vi "gpibListener.vi"() -> ()   [LabVIEW 2011]
panel:
  in  "stop":bool
  out "Error Code":i32
  out "Error Status":bool
  out "Error Source":string
  in  "VISA resource name":refnum<visa-resource-name>
  out "Read Value":string
  out "Bytes Read":dbl
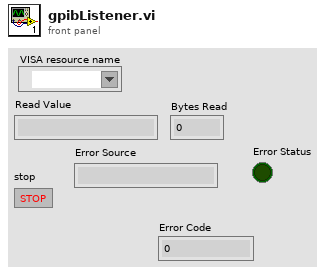
[diagram p1: front panel]
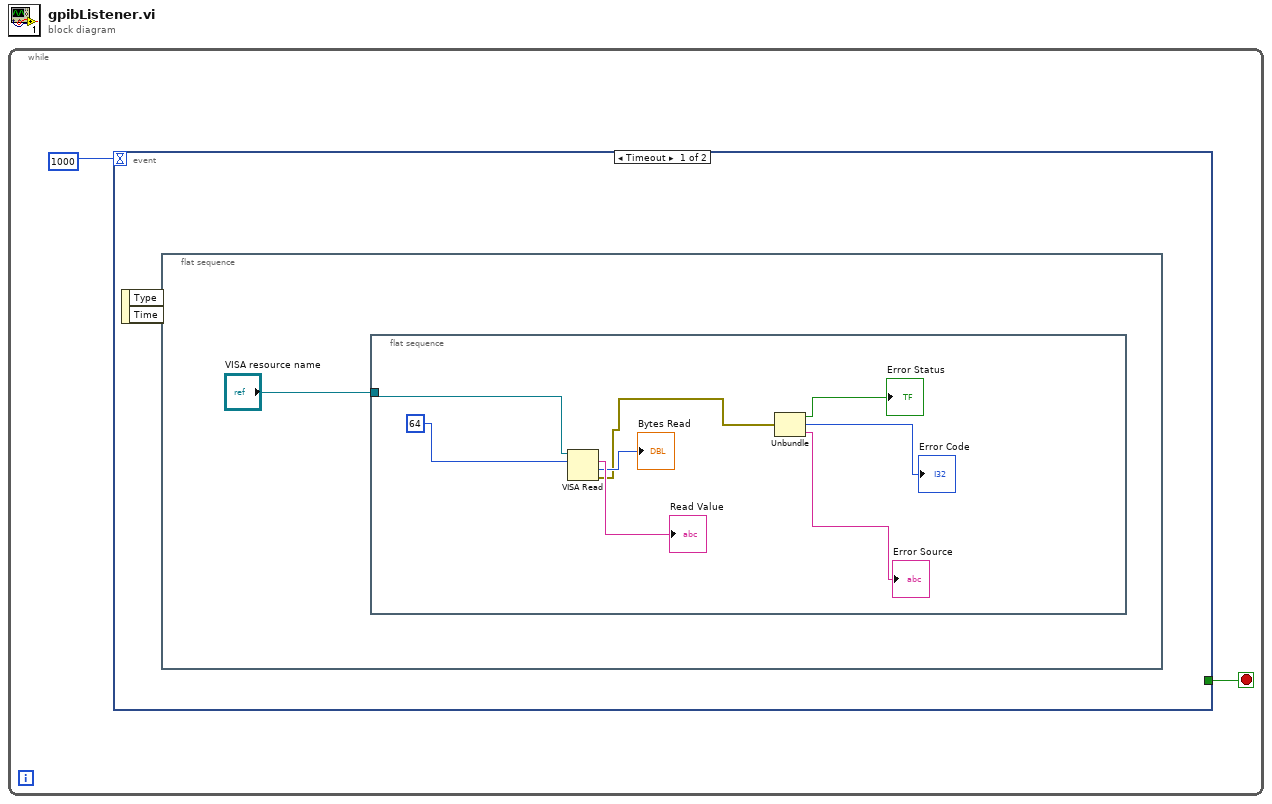
[diagram p0: block diagram]
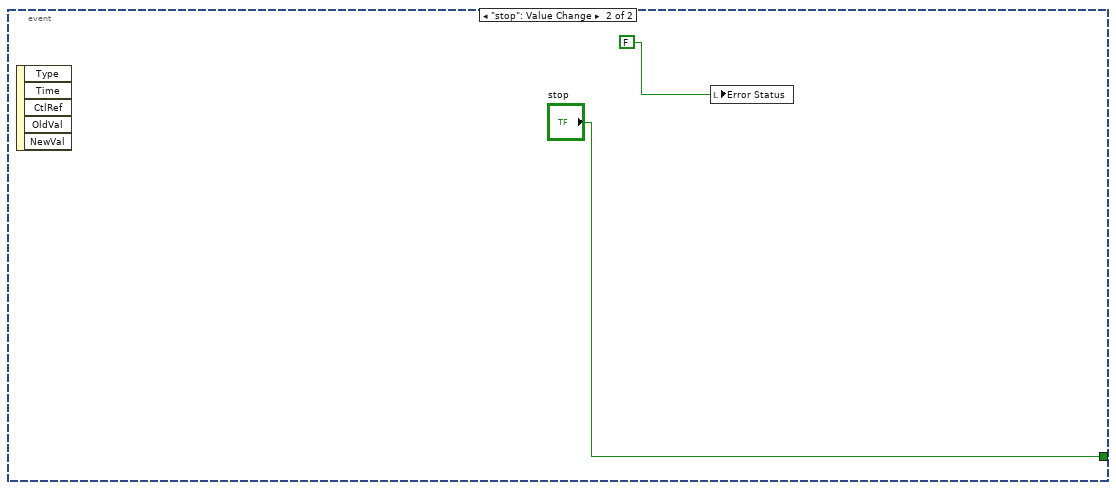
[diagram p2: hidden frame]
diagram:
  n1 = while {
    stop <- w1 stop-if-true
    n2 = event shown="[0] Timeout" {
      selector: _ -> [_ _]
      dyn-events: _ -> [_ _]
      timeout: 1000 -> [_ _]
      tunnel: [_ "stop"] -> w1
      event Timeout {
        n3 = event-data() -> ()  [unwired: 1 in, 2 out]
        n4 = flat-sequence {
          frame #0 {
            n5 = flat-sequence {
              tunnel: "VISA resource name" -> [w8]
              frame #0 {
                n6 = VISA Read(VISA resource name=w8, byte count=64) -> (read buffer=→"Read Value":string, return count=→"Bytes Read":u32, error out=w7:errorcluster)  [unwired: 1 in, 1 out]
                n7 = Unbundle(w7) -> ("status"=→"Error Status":bool, "code"=→"Error Code":i32, "source"=→"Error Source":string)
              }
            }
          }
        }
      }
      event "stop": Value Change {
        n8 = event-data() -> ()  [unwired: 1 in, 5 out]
        n9 = local write "Error Status"(FALSE) -> ()
      }
    }
  }
